vi "PCO_GetVersion_SDK.vi"(1 "pszNameIn":string, 7 "error in (no error)":errorcluster {"code" format="%x"}) -> (21 "pszName":string, 22 "piMajor":i32, 23 "piMinor":i32, 24 "piPatch":i32, 25 "piBuild":i32, 26 "ErrorMessage":i32 format="%x", 27 "error out":errorcluster {"code" format="%x"})   [LabVIEW 2019, in "SDK.lvlib" / "CameraAccess.lvlib"]
doc: "Returns information about the current sc2_cam, or the sc2_cam interface library version."
uses:
  CameraAccess.lvlib
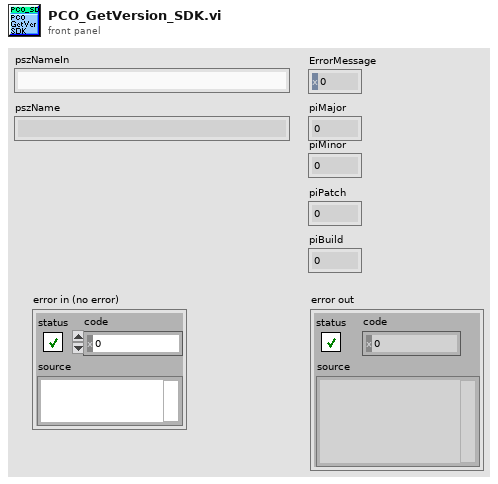
[diagram p1: front panel]
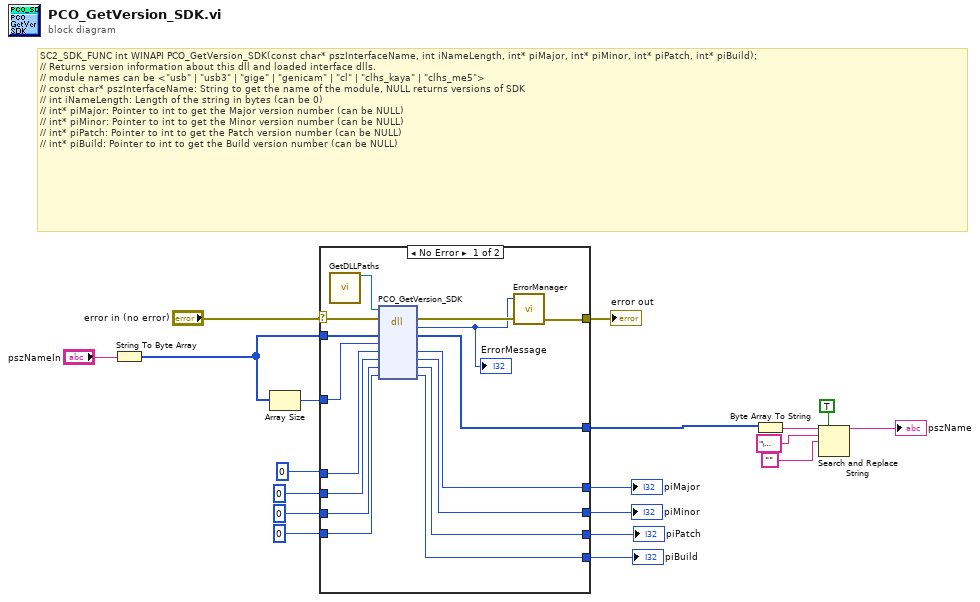
[diagram p0: block diagram]
diagram:
  # "SC2_SDK_FUNC int WINAPI PCO_GetVersion_SDK(const char* pszInterfaceName, int iNameLength, int* piMajor, int* piMinor, int* piPatch, int* piBuild);\n// Returns version information about this dll and loaded interface dlls.\n// module names can be <\"usb\" | \"usb3\" | \"gige\" | \"genicam\" | \"cl\" | \"clhs_kaya\" | \"clhs_me5\">\n// const char* pszInterfaceName: String to get the name of the module, NULL returns versions of SDK\n// int iNameLength: Length of the string in bytes (can be 0)\n// int* piMajor: Pointer to int to get the Major version number (can be NULL)\n// int* piMinor: Pointer to int to get the Minor version number (can be NULL)\n// int* piPatch: Pointer to int to get the Patch version number (can be NULL)\n// int* piBuild: Pointer to int to get the Build version number (can be NULL)"
  n1 = String To Byte Array(string="pszNameIn") -> (unsigned byte array=w2:u8[])
  n2 = Array Size(array=w2) -> (size(s)=w3:i32)
  n3 = case shown="No Error" "error in (no error)" {
    selector: "error in (no error)" -> [w33 w41]
    tunnel: [w20 w36] -> w4
    tunnel: [w34 w41] -> w19
    tunnel: [w31 w38] -> w17
    tunnel: [w30 w40] -> w16
    tunnel: [w29 w39] -> w15
    tunnel: w3 -> [w28 _]
    tunnel: 0 ("piMinor") -> [w27 w40]
    tunnel: 0 ("build") -> [w26 w39]
    tunnel: 0 ("piMinor") -> [w25 w38]
    tunnel: [w24 w37] -> w7
    tunnel: 0 ("piPatch") -> [w23 w37]
    tunnel: w2 -> [w21 w36]
    frame No Error {
      n4 = call "GetDLLPaths.vi"() -> ("SC2_Cam_Path"=w22:path)  [unwired: 8 in, 3 out]
      n5 = dll-call lib="?" fn="PCO_GetVersion_SDK"(path in=w22, error in=w33, "pszInterfaceName"=w21, "iNameLength"=w28, "piMajor"=w25, "piMinor"=w27, "piPatch"=w23, "piBuild"=w26) -> (error out=w35:errorcluster, "return type"=w32:i32, "pszInterfaceName"=w20:u8[], "piMajor"=w31:i32, "piMinor"=w30:i32, "piPatch"=w24:i32, "piBuild"=w29:i32)  [unwired: 2 in, 1 out]
      "ErrorMessage" <- w32
      n6 = call "ErrorManager.vi"("error in (no error)"=w35, "error code"=w32) -> ("error out"=w34:errorcluster)  [unwired: 2 in, 1 out]
    }
    frame Error {
    }
  }
  "error out" <- w19
  "piMajor" <- w17
  "piMinor" <- w16
  "piBuild" <- w15
  "piPatch" <- w7
  n7 = Byte Array To String(unsigned byte array=w4) -> (string=w12:string)
  n8 = Search and Replace String(replace all?=TRUE ("replace all? (F)"), input string=w12, search string="\u0000", replace string="" ("replace string (\"\")")) -> (result string=→"pszName":string)  [unwired: 4 in, 3 out]
